vi "Initialize.vi"() -> ()   [LabVIEW 2013]
uses:
  libtiepie.dll
panel:
  out "InitializeADCcard_output":T1
  in  "InitializeADCcard_input":T2={"Sample Frequency/Hz"=200000000, "Record Length/Samples"=50000, "CH1_Coupling"=1, "Channel 1_Range"=4.0, "a0"=-0.25, "a1"=0.0064, "a2"=1.8e-05} {"Channel 1_Range" items=["80 V"=80.0, "40 V"=40.0, "20 V"=20.0, "8 V"=8.0, "4 V"=4.0, "2 V"=2.0, "800 mV"=0.8, "400 mV"=0.4, "200 mV"=0.2]; "CH1_Coupling" items=["Volt DC"=1, "Volt AC"=2, "Ampere DC"=4, "Ampere AC"=8, "Ohm"=16]}
  out "channelCount":u16
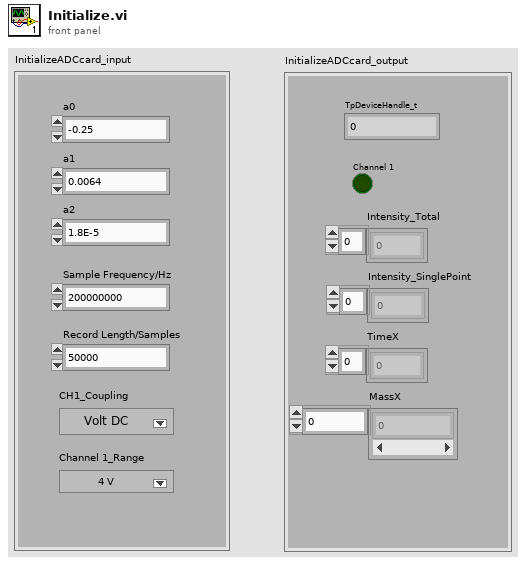
[diagram p1: front panel]
types:
  T1 = cluster{"TpDeviceHandle_t":u32, "Channel 1":bool, "Intensity_SinglePoint":sgl[], "Intensity_Total":sgl[], "TimeX":dbl[], "MassX":dbl[]}
  T2 = cluster{"Sample Frequency/Hz":i32, "Record Length/Samples":u64, "CH1_Coupling":u64, "Channel 1_Range":dbl, "a0":dbl, "a1":dbl, "a2":dbl}
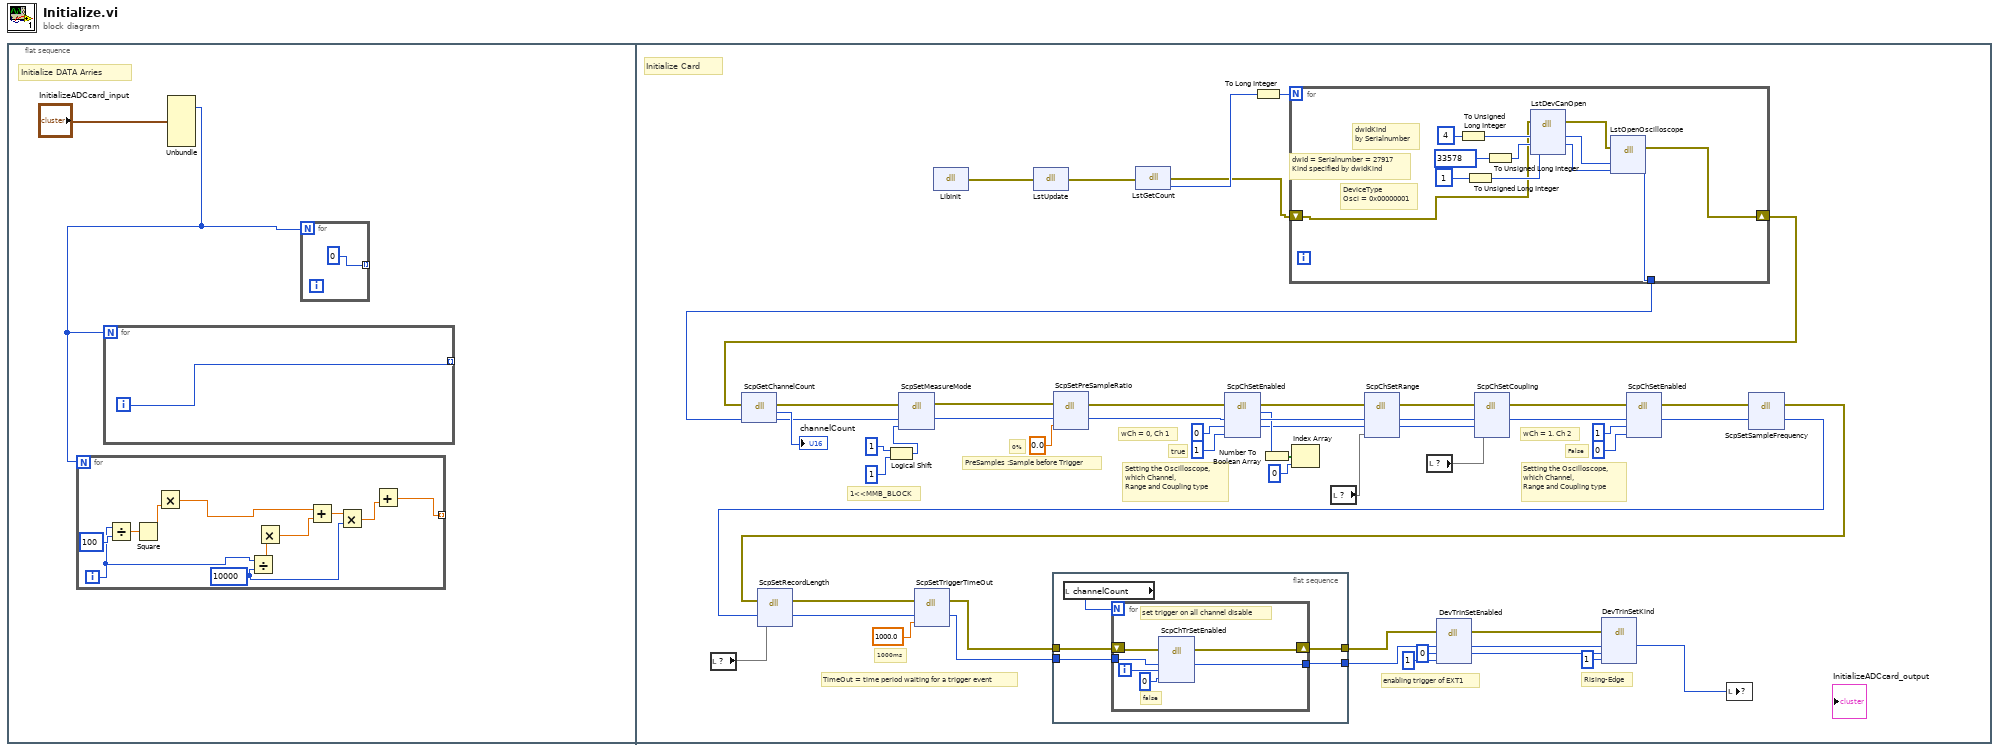
[diagram p0: block diagram]
diagram:
  n1 = flat-sequence {
    frame #0 {
      # "Initialize DATA Arries"
      n2 = Unbundle("InitializeADCcard_input") -> ("Record Length/Samples"=w1:u64)  [unwired: 6 out]
      n3 = for {
        N: w1 -> [_]
        tunnel: [w9] -> w4 mode=indexing
        i -> [w13]
        w7 = 10000
        n4 = Divide(x=w13, y=100) -> (x/y=w16:dbl)
        n5 = Square(x=w16) -> (x^2=w18:dbl)
        n6 = Multiply(y=w18) -> (x*y=w12:dbl)  [unwired: 1 in]
        n7 = Divide(x=w13, y=w7) -> (x/y=w14:dbl)
        n8 = Multiply(y=w14) -> (x=w17:dbl, x*y=w11:dbl)
        n9 = Add(x=w12, y=w11) -> (x+y=w8:dbl)
        n10 = Multiply(x=w8, y=w7) -> (x*y=w6:dbl)
        n11 = Add(y=w6) -> (x=w10:dbl, x+y=w9:dbl)
      }
      n12 = for {
        N: w1 -> [_]
        tunnel: [w19] -> w5 mode=indexing
        i -> [w19]
      }
      n13 = for {
        N: w1 -> [_]
        tunnel: [0] -> w3 mode=indexing
      }
    }
    frame #1 {
      # "Rising-Edge"
      # "enabling trigger of EXT1"
      # "1000ms"
      # "TimeOut = time period waiting for a trigger event"
      # "Setting the Oscilloscope,\nwhich Channel, \nRange and Coupling type"
      # "wCh = 1. Ch 2"
      # "False"
      # "Setting the Oscilloscope,\nwhich Channel, \nRange and Coupling type"
      # "wCh = 0, Ch 1"
      # "true"
      # "0%"
      # "PreSamples :Sample before Trigger"
      # "1<<MMB_BLOCK"
      # "Initialize Card"
      n14 = local read item#-1() -> (w21)
      n15 = Logical Shift(y=u32 1, x=u32 1 ("y")) -> (x << y=w48:u32)
      n16 = dll-call lib="PTH1Fabs CUsers82158DesktopTOF software\t数据卡\nlibtiepie.dll" fn="LibInit"() -> (error out=w74:errorcluster)  [unwired: 4 in, 1 out]
      n17 = dll-call lib="PTH1Fabs CUsers82158DesktopTOF software\t数据卡\nlibtiepie.dll" fn="LstUpdate"(error in=w74) -> (error out=w26:errorcluster)  [unwired: 3 in, 1 out]
      n18 = flat-sequence {
        tunnel: w32 -> [w80]
        tunnel: w33 -> [w79]
        tunnel: [w77] -> w41
        tunnel: [w76] -> w42
        frame #0 {
          n19 = local read "channelCount"() -> (w78:u16)
          n20 = for {
            N: w78 -> [_]
            tunnel: w80 -> [w83]
            shift-right: [w82] -> w77
            shift-left: w79 -> [w84]
            tunnel: [w81] -> w76
            i -> [w86]
            # "set trigger on all channel disable"
            # "false"
            n21 = dll-call lib="PTH1Fabs CUsers82158DesktopTOF software\t数据卡\nlibtiepie.dll" fn="ScpChTrSetEnabled"(error in=w84, "TpDeviceHandle_t"=w83, "wCh"=w86, "bEnable"=u8 0) -> (error out=w82:errorcluster, "TpDeviceHandle_t"=w81:u32)  [unwired: 5 in, 1 out]
          }
        }
      }
      n22 = dll-call lib="PTH1Fabs CUsers82158DesktopTOF software\t数据卡\nlibtiepie.dll" fn="LstGetCount"(error in=w26) -> (error out=w27:errorcluster, "Count"=w28:u32)  [unwired: 2 in, 1 out]
      n23 = To Long Integer(number=w28) -> (32bit integer=w75:i32)
      n24 = for {
        N: w75 -> [_]
        shift-right: [w89] -> w31
        shift-left: w27 -> [w88]
        tunnel: [w87] -> w30
        # "DeviceType\nOsci = 0x00000001"
        # "dwId = Serialnumber = 27917\nKind specified by dwIdKind"
        # "dwIdKind\nby Serialnumber"
        n25 = To Unsigned Long Integer(number=4) -> (unsigned 32bit integer=w97:u32)
        n26 = To Unsigned Long Integer(number=1) -> (unsigned 32bit integer=w95:u32)
        n27 = To Unsigned Long Integer(number=33578) -> (unsigned 32bit integer=w93:u32)
        n28 = dll-call lib="PTH1Fabs CUsers82158DesktopTOF software\t数据卡\nlibtiepie.dll" fn="LstDevCanOpen"(error in=w88, "dwIdKind"=w97, "dwId"=w93, "dwDeviceType"=w95) -> (error out=w90:errorcluster, "dwIdKind"=w91:u32, "dwId"=w92:u32)  [unwired: 4 in, 1 out]
        n29 = dll-call lib="PTH1Fabs CUsers82158DesktopTOF software\t数据卡\nlibtiepie.dll" fn="LstOpenOscilloscope"(error in=w90, "dwIdKind"=w91, "dwId"=w92) -> (error out=w89:errorcluster, "TpDeviceHandle_t"=w87:u32)  [unwired: 4 in, 1 out]
      }
      n30 = dll-call lib="PTH1Fabs CUsers82158DesktopTOF software\t数据卡\nlibtiepie.dll" fn="ScpGetChannelCount"(error in=w31, "TpDeviceHandle_t"=w30) -> (error out=w44:errorcluster, "channelCount"=→"channelCount":u16, "TpDeviceHandle_t"=w43:u32)  [unwired: 2 in, 1 out]
      n31 = dll-call lib="PTH1Fabs CUsers82158DesktopTOF software\t数据卡\nlibtiepie.dll" fn="ScpSetMeasureMode"(error in=w44, "TpDeviceHandle_t"=w43, "dwMeasureMode"=w48) -> (error out=w54:errorcluster, "TpDeviceHandle_t"=w55:u32)  [unwired: 4 in, 1 out]
      n32 = dll-call lib="PTH1Fabs CUsers82158DesktopTOF software\t数据卡\nlibtiepie.dll" fn="ScpSetPreSampleRatio"(error in=w54, "TpDeviceHandle_t"=w55, "dPreSampleRatio"=0.0) -> (error out=w50:errorcluster, "TpDeviceHandle_t"=w52:u32)  [unwired: 4 in, 1 out]
      n33 = dll-call lib="PTH1Fabs CUsers82158DesktopTOF software\t数据卡\nlibtiepie.dll" fn="ScpChSetEnabled"(error in=w50, "TpDeviceHandle_t"=w52, "wCh"=u16 0, "bEnable"=u8 1) -> (error out=w59:errorcluster, "Enabled"=w66:u8, "TpDeviceHandle_t"=w67:u32, "wCh"=w60:u16)  [unwired: 3 in, 1 out]
      n34 = Number To Boolean Array(number=w66) -> (Boolean array=w64:bool[])
      n35 = Index Array(array=w64, index=0) -> ()  [unwired: 1 out]
      n36 = local read item#-1() -> (w63)
      n37 = dll-call lib="PTH1Fabs CUsers82158DesktopTOF software\t数据卡\nlibtiepie.dll" fn="ScpChSetRange"(error in=w59, "TpDeviceHandle_t"=w67, "wCh"=w60, "dRange"=w63) -> (error out=w68:errorcluster, "TpDeviceHandle_t"=w70:u32, "wCh"=w69:u16)  [unwired: 4 in, 1 out]
      n38 = local read item#-1() -> (w62)
      n39 = dll-call lib="PTH1Fabs CUsers82158DesktopTOF software\t数据卡\nlibtiepie.dll" fn="DevTrInSetEnabled"(error in=w41, "hDevice"=w42, "wInput"=u16 0, "enable"=u8 1) -> (error out=w38:errorcluster, "hDevice"=w37:u32, "wInput"=w36:u16)  [unwired: 4 in, 1 out]
      n40 = dll-call lib="PTH1Fabs CUsers82158DesktopTOF software\t数据卡\nlibtiepie.dll" fn="ScpChSetCoupling"(error in=w68, "TpDeviceHandle_t"=w70, "wCh"=w69, "qwCoupling"=w62) -> (error out=w51:errorcluster, "TpDeviceHandle_t"=w73:u32)  [unwired: 5 in, 1 out]
      n41 = dll-call lib="PTH1Fabs CUsers82158DesktopTOF software\t数据卡\nlibtiepie.dll" fn="DevTrInSetKind"(error in=w38, "hDevice"=w37, "wInput"=w36, "qwkind"=u64 1) -> ("hDevice"=w29:u32)  [unwired: 5 in, 2 out]
      n42 = dll-call lib="PTH1Fabs CUsers82158DesktopTOF software\t数据卡\nlibtiepie.dll" fn="ScpChSetEnabled"(error in=w51, "TpDeviceHandle_t"=w73, "wCh"=u16 1, "bEnable"=u8 0) -> (error out=w56:errorcluster, "TpDeviceHandle_t"=w57:u32)  [unwired: 5 in, 1 out]
      n43 = local write item#-1(w29) -> ()
      n44 = dll-call lib="PTH1Fabs CUsers82158DesktopTOF software\t数据卡\nlibtiepie.dll" fn="ScpSetSampleFrequency"(error in=w56, "TpDeviceHandle_t"=w57) -> (error out=w23:errorcluster, "TpDeviceHandle_t"=w22:u32, "SampleFrequency"=w53:dbl)  [unwired: 4 in, 1 out]
      n45 = dll-call lib="PTH1Fabs CUsers82158DesktopTOF software\t数据卡\nlibtiepie.dll" fn="ScpSetRecordLength"(error in=w23, "TpDeviceHandle_t"=w22, "qwRecordLength"=w21) -> (error out=w25:errorcluster, "TpDeviceHandle_t"=w24:u32)  [unwired: 4 in, 1 out]
      n46 = dll-call lib="PTH1Fabs CUsers82158DesktopTOF software\t数据卡\nlibtiepie.dll" fn="ScpSetTriggerTimeOut"(error in=w25, "TpDeviceHandle_t"=w24, "dTimeOut"=1000.0) -> (error out=w33:errorcluster, "TpDeviceHandle_t"=w32:u32)  [unwired: 4 in, 1 out]
    }
  }
